vi "Init LCD.vi"(8 "error in (no error)":errorcluster, 11 "Refnum in":refnum<k20>) -> (0 "error out":errorcluster, 3 "Refnum out":refnum<k20>)   [LabVIEW 2013]
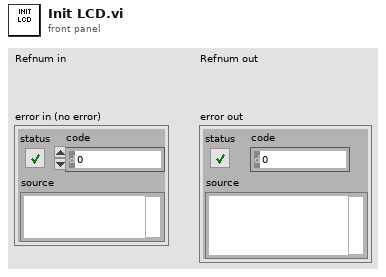
[diagram p1: front panel]
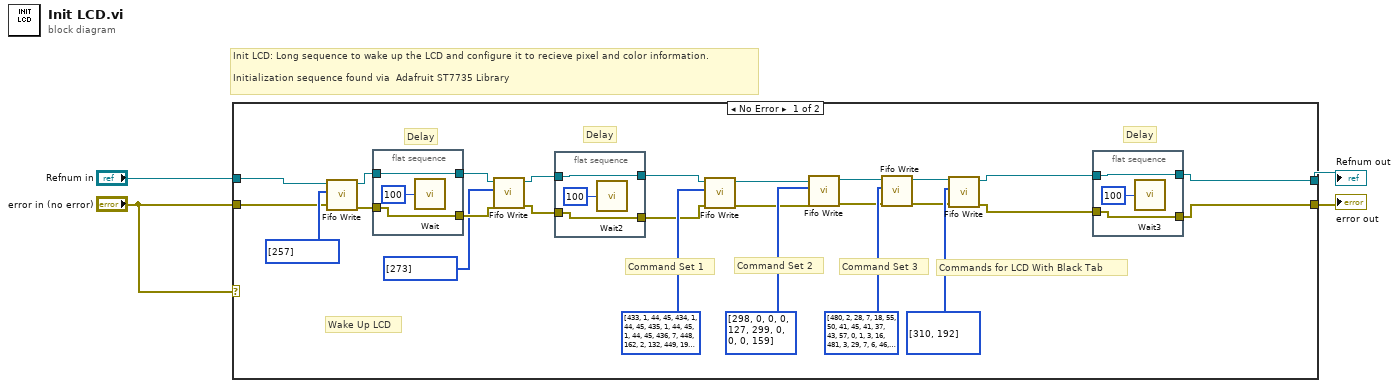
[diagram p0: block diagram]
diagram:
  # "Init LCD: Long sequence to wake up the LCD and configure it to recieve pixel and color information.\n\nInitialization sequence found via  Adafruit ST7735 Library"
  n1 = case shown="No Error" "error in (no error)" {
    tunnel: [w5 w40] -> w4
    tunnel: [w6 w41] -> w3
    tunnel: "error in (no error)" -> [w18 w40]
    tunnel: "Refnum in" -> [w19 w41]
    frame No Error {
      # "Wake Up LCD"
      # "Delay"
      # "Delay"
      # "Delay"
      # "Commands for LCD With Black Tab"
      # "Command Set 3"
      # "Command Set 2"
      # "Command Set 1"
      n2 = call "Fifo Write.vi"("error in (no error)"=w18, "Data"=u16[] [257], "Refnum in"=w19) -> ("error out"=w16:errorcluster, "Refnum out"=w17:refnum<k20>)  [unwired: 7 in]
      n3 = flat-sequence {
        tunnel: w17 -> [w38]
        tunnel: w16 -> [w37]
        tunnel: [w38] -> w15
        tunnel: [w37] -> w14
        frame #0 {
          n4 = call "Wait"("Count(mSec)"=u32 100) -> ()  [unwired: 1 out]
        }
      }
      n5 = call "Fifo Write.vi"("error in (no error)"=w14, "Data"=u16[] [273], "Refnum in"=w15) -> ("error out"=w11:errorcluster, "Refnum out"=w12:refnum<k20>)  [unwired: 7 in]
      n6 = flat-sequence {
        tunnel: w12 -> [w35]
        tunnel: w11 -> [w34]
        tunnel: [w35] -> w10
        tunnel: [w34] -> w9
        frame #0 {
          n7 = call "Wait2"("Count(mSec)"=u32 100) -> ()  [unwired: 1 out]
        }
      }
      n8 = call "Fifo Write.vi"("error in (no error)"=w9, "Data"=u16[] [433, 1, 44, 45, 434, 1, 44, 45, 435, 1, 44, 45, 1, 44, 45, 436, 7, 448, 162, 2, 132, 449, 197, 450, 10, 0, 451, 138, 42, 452, 138, 238, 453, 14, 288, 310, 200, 314, 5], "Refnum in"=w10) -> ("error out"=w22:errorcluster, "Refnum out"=w23:refnum<k20>)  [unwired: 7 in]
      n9 = call "Fifo Write.vi"("error in (no error)"=w22, "Data"=u16[] [298, 0, 0, 0, 127, 299, 0, 0, 0, 159], "Refnum in"=w23) -> ("error out"=w25:errorcluster, "Refnum out"=w24:refnum<k20>)  [unwired: 7 in]
      n10 = call "Fifo Write.vi"("error in (no error)"=w25, "Data"=u16[] [480, 2, 28, 7, 18, 55, 50, 41, 45, 41, 37, 43, 57, 0, 1, 3, 16, 481, 3, 29, 7, 6, 46, 44, 41, 45, 46, 46, 55, 63, 0, 0, 2, 16, 275, 297], "Refnum in"=w24) -> ("error out"=w27:errorcluster, "Refnum out"=w26:refnum<k20>)  [unwired: 7 in]
      n11 = call "Fifo Write.vi"("error in (no error)"=w27, "Data"=u16[] [310, 192], "Refnum in"=w26) -> ("error out"=w7:errorcluster, "Refnum out"=w8:refnum<k20>)  [unwired: 7 in]
      n12 = flat-sequence {
        tunnel: w8 -> [w32]
        tunnel: w7 -> [w31]
        tunnel: [w32] -> w6
        tunnel: [w31] -> w5
        frame #0 {
          n13 = call "Wait3"("Count(mSec)"=u32 100) -> ()  [unwired: 1 out]
        }
      }
    }
    frame Error {
    }
  }
  "error out" <- w4
  "Refnum out" <- w3
